vi "CM_WriteVelocities.vi"(8 "error in":errorcluster, 11 "Velocities":dbl[](array[numeric])) -> (0 "error out":errorcluster)   [LabVIEW 2016]
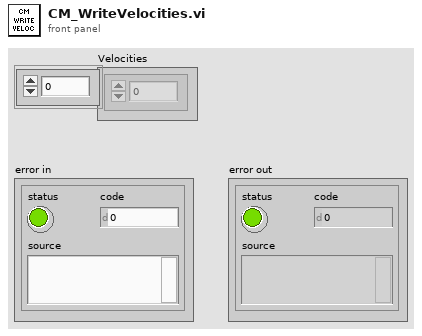
[diagram p1: front panel]
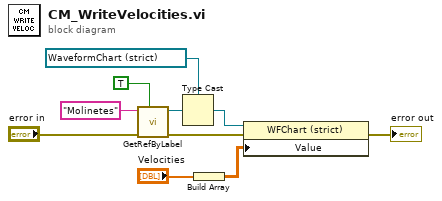
[diagram p0: block diagram]
diagram:
  n1 = call "GetRefByLabel.vi"("InsideTab"=TRUE, "error in"="error in", "Label"="Molinetes") -> ("error out"=w2:errorcluster, "Ctl Refnum"=w6:refnum<vi>)  [unwired: 6 in, 1 out]
  n2 = Type Cast(type=refnum<vi> refnum ("Grupo 1"), x=w6) -> (*(type *) &x=w5:refnum<vi>)
  n3 = Build Array("Velocities") -> (w4:dbl[][])
  n4 = property class="WFChart (strict)"(reference=w5, error in=w2, "Value"=w4) -> (error out=→"error out":errorcluster)  [unwired: 1 out]
